vi "Read an analog IO desc.vi"(7 "Variable Defenition":T1={"ID"=0, "Name"="HVPSU Head Voltage", "Quantity"=enum."Torque", "Unit"="", "Maximum upd"=enum."2 Hz", "Comment"="Var Common", "Help file Name"="HVPSU Head Voltage", "Help file Section "="", "Category"=enum."No Category", "User adjustable Scaling"=FALSE, "Default Scaling"={"Gain"=1.0, "Offset"=0.0}, "In use"=FALSE, "Default Unit"=0} {"Default Scaling"."Offset" format="%.5f"; "Default Scaling"."Gain" format="%.5f"}) -> (4 "Header":string, 8 "concatenated string":string)   [LabVIEW 2011]
uses:
  Measurments Handling/Fixed Analog Channel Definition.ctl
  Measurments Handling/Units/Quantity enum.ctl
  Measurments Handling/Update frequensies.ctl
  Measurments Handling/Channel catagory Enum.ctl
  Measurments Handling/Scaling.ctl
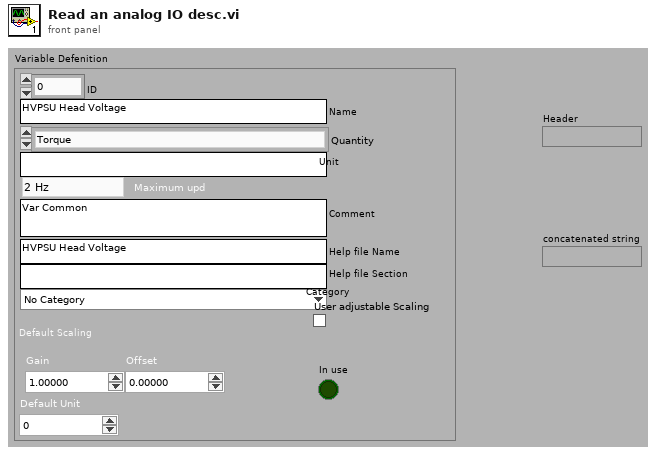
[diagram p1: front panel]
types:
  T1 = typedef "Fixed Analog Channel Definition.ctl" = cluster{"ID":u16, "Name":string, "Quantity":T2, "Unit":string, "Maximum upd":T3, "Comment":string, "Help file Name":string, "Help file Section ":string, "Category":T4, "User adjustable Scaling":bool, "Default Scaling":T5, "In use":bool, "Default Unit":i32}
  T2 = typedef "Quantity enum.ctl" = enum16{"Acceleration", "Angle", "Current", "Force", "Distance", "Pressure", "Resistance", "Rotational Speed", "Speed", "Temperature", "Tension", "Torque", "Voltage", "Weight"}
  T3 = typedef "Update frequensies.ctl" = enum16{"2 Hz", "1 Hz", "0.1 Hz"}
  T4 = typedef "Channel catagory Enum.ctl" = enum16{"No Category", "Power", "Temperature", "Pressure"}
  T5 = typedef "Scaling.ctl" = cluster{"Gain":dbl, "Offset":dbl}
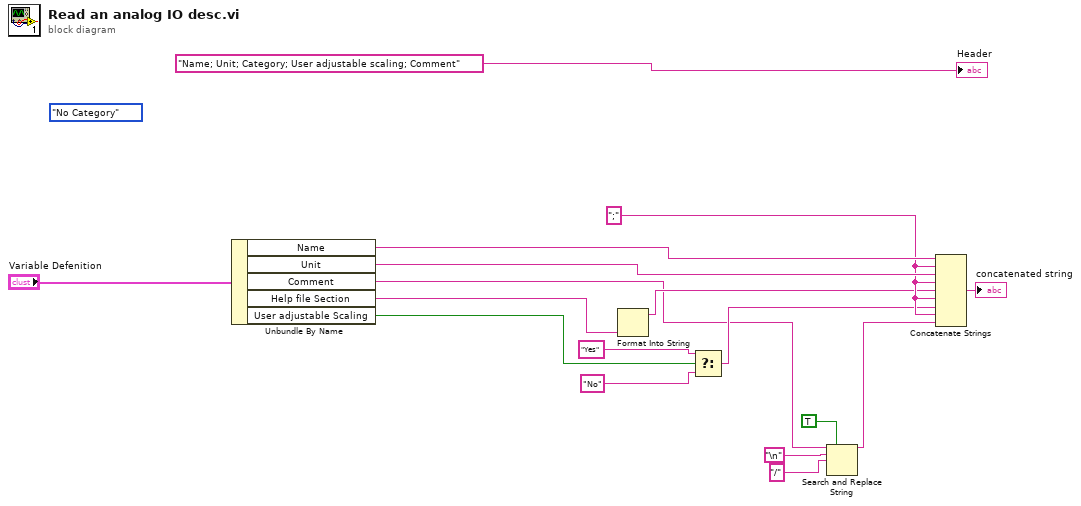
[diagram p0: block diagram]
diagram:
  (unwired) Channel_catagory_Enum."No Category" ("Catagory")
  w13 = ";" ("string")
  n1 = Unbundle By Name("Variable Defenition") -> ("Name"=w16:string, "Unit"=w15:string, "Comment"=w2:string, "Help file Section"=w14:string, "User adjustable Scaling"=w12:bool)
  n2 = Format Into String(w14) -> (resulting string=w9:string)  [unwired: 3 in, 1 out]
  n3 = Select(t="Yes" ("string"), s=w12, f="No" ("string")) -> (s? t:f=w8:string)
  n4 = Search and Replace String(replace all?=TRUE ("replace all? (F)"), input string=w2, search string="\n", replace string="/" ("replace string (\"\")")) -> (result string=w1:string)  [unwired: 4 in, 3 out]
  n5 = Concatenate Strings(w16, w13, w15, w13, w9, w13, w8, w13, w1) -> (→"concatenated string":string)
  "Header" <- "Name; Unit; Category; User adjustable scaling; Comment" ("Header")
